vi "Init.vi"(8 "error in (no error)":errorcluster, 11 "Simulada in":refnum<class "Simulada.lvclass">) -> (0 "error out":errorcluster, 3 "Simulada out":refnum<class "Simulada.lvclass">)   [LabVIEW 2020, in "Simulada.lvclass"]
uses:
  Simulada.lvclass
  Abstract/Serial Device/Serial Device.lvclass
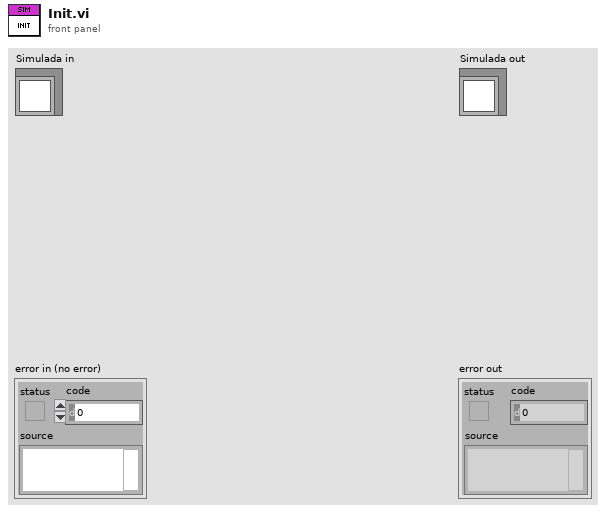
[diagram p1: front panel]
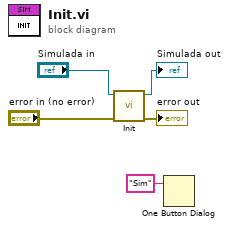
[diagram p0: block diagram]
diagram:
  n1 = call-parent "Init.vi"("error in (no error)"="error in (no error)", "Serial Device in"="Simulada in") -> ("error out"=→"error out":errorcluster, "Serial Device out"=→"Simulada out":refnum<class "Simulada.lvclass">)  [unwired: 8 in]
  n2 = One Button Dialog(message="Sim") -> ()  [unwired: 1 in, 1 out]
